vi "RunningCounter with Reset_2016.vi"(7 "Reset?":bool, 8 "INC?":bool, 11 "rollover":u64) -> (0 "rollover":bool, 3 "count":u64)   [LabVIEW 2016]
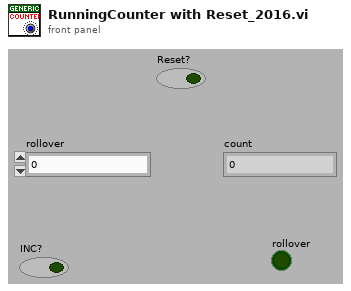
[diagram p1: front panel]
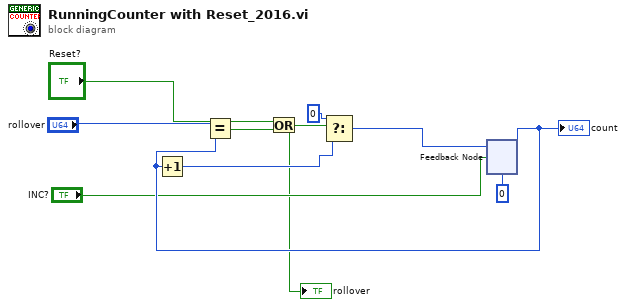
[diagram p0: block diagram]
diagram:
  n1 = feedback #1(u64 0) -> (w6:u64)
  "count" <- w6
  n2 = Increment(x=w6) -> (x+1=w8:u64)
  n3 = Equal?(x="rollover", y=w6) -> (x = y?=w2:bool)
  n4 = Or(x="Reset?", y=w2) -> (x .or. y?=w3:bool)
  "rollover" <- w3
  n5 = Select(t=u64 0, s=w3, f=w8) -> (s? t:f=w5:u64)
  n6 = feedback-in #1(w5, "INC?") -> ()
